vi "BMark_OpenWindow.vi"(6 "Graveyward Position Key":string="Eulogy.Graveyard.Position", 8 "Error In":errorcluster, 11 "Graveyard Window In":refnum<vi>) -> (0 "Error Out":errorcluster, 2 "Bounds":T1, 3 "Graveyward Window Out":refnum<vi>)   [LabVIEW 2018, in "Bookmark Manager.lvlib"]
uses:
  Bookmark Manager.lvlib
  <resource>/dialog/lvconfig.llb/LV Config Read String.vi
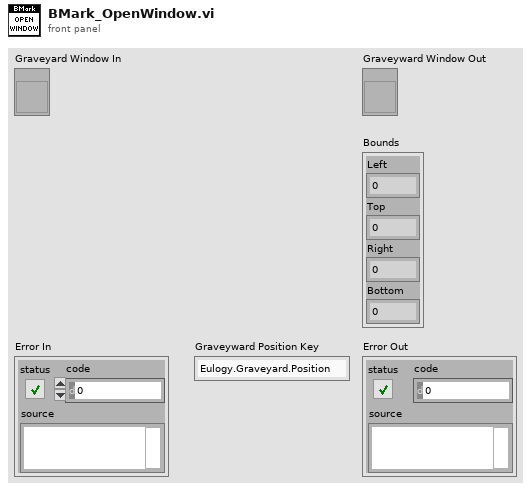
[diagram p1: front panel]
types:
  T1 = cluster{"Left":i16, "Top":i16, "Right":i16, "Bottom":i16}
  T2 = enum32{"Invalid", "Standard", "Closed", "Hidden", "Minimized", "Maximized"}
  T3 = typedef "LVAllMonitorsDisplayTypeDef.ctl" = cluster{"Bounds":cluster{"Left":i16, "Top":i16, "Right":i16, "Bottom":i16}, "Depth":i16}[]
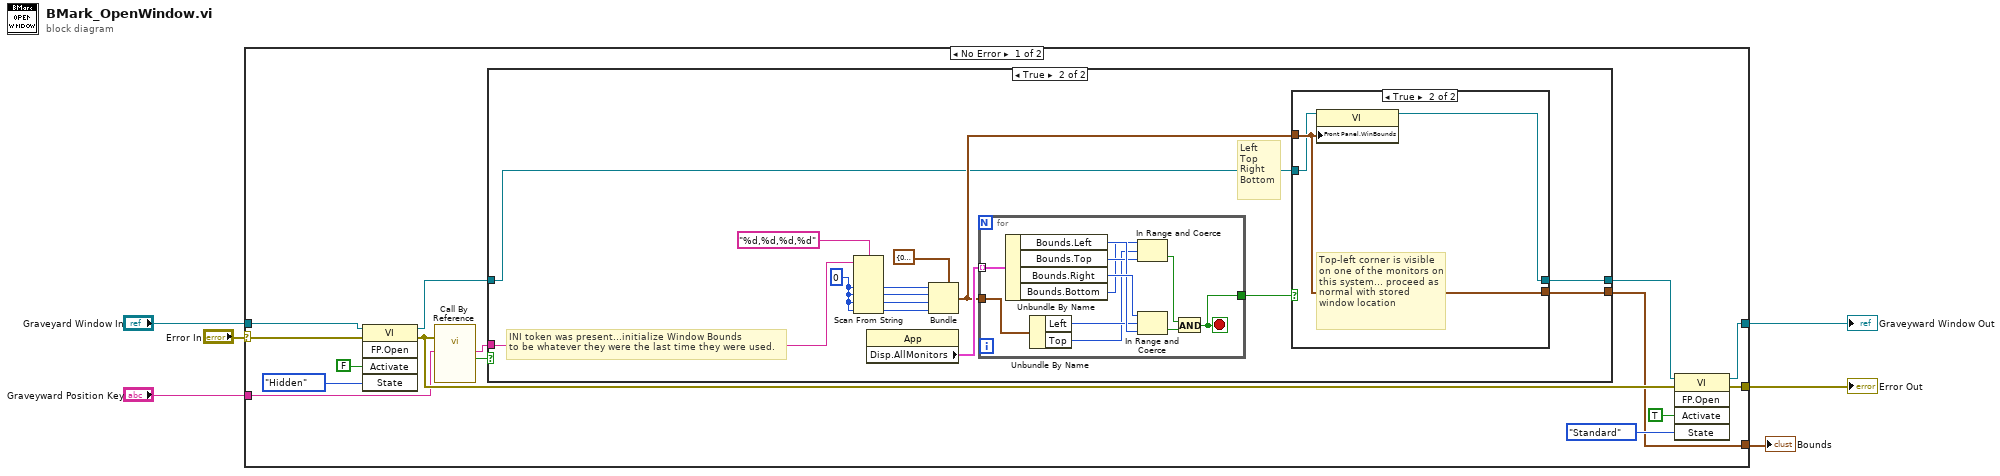
[diagram p0: block diagram]
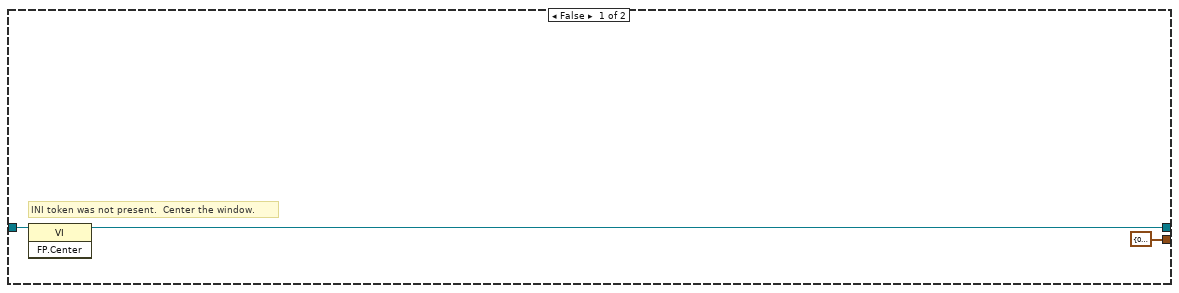
[diagram p2: hidden frame]
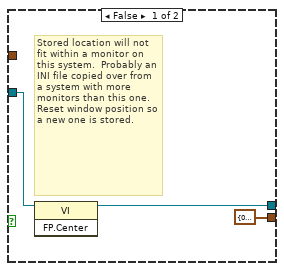
[diagram p3: hidden frame]
diagram:
  n1 = case shown="No Error" "Error In" {
    selector: "Error In" -> [w8 w57]
    tunnel: "Graveyard Window In" -> [w19 w56]
    tunnel: [w12 w56] -> w5
    tunnel: [w11 w57] -> w4
    tunnel: [w9 _] -> w3
    tunnel: "Graveyward Position Key" -> [w7 _]
    frame No Error {
      n2 = invoke class="VI" method="FP.Open"(reference=w19, error in=w8, "Activate"=FALSE ("Activate?"), "State"=T2."Hidden") -> (reference out=w14:refnum<vi>, error out=w10:errorcluster)  [unwired: 1 in, 3 out]
      n3 = call-by-ref "?"(error in=w10, "key"=w7) -> ("found?"=w15:bool, "value"=w16:string)  [unwired: 5 in, 3 out]
      n4 = case shown="True" w15 {
        tunnel: [T1 {"Left"=0, "Top"=0, "Right"=0, "Bottom"=0} ("Front Panel.PanelBounds") w27] -> w9
        tunnel: w16 -> [_ w38]
        tunnel: w14 -> [w23 w26]
        tunnel: [w22 w25] -> w13
        frame False {
          # "INI token was not present.  Center the window."
          n5 = invoke class="VI" method="FP.Center"(reference=w23) -> (reference out=w22:refnum<vi>)  [unwired: 2 in, 2 out]
        }
        frame True {
          w36 = i16 0 ("default value 1")
          # "Left\nTop\nRight\nBottom"
          # "INI token was present...initialize Window Bounds\nto be whatever they were the last time they were used."
          n6 = Scan From String(format string="%d,%d,%d,%d", input string=w38, default 1=w36, default 2=w36, default 3=w36, default 4=w36) -> (output 1=w35:i16, output 2=w34:i16, output 3=w33:i16, output 4=w32:i16)  [unwired: 2 in, 3 out]
          n7 = property class="App"() -> ("Disp.AllMonitors"=w30:T3)  [unwired: 2 in, 2 out]
          n8 = Bundle(cluster=T1 {"Left"=0, "Top"=0, "Right"=0, "Bottom"=0} ("Front Panel.PanelBounds"), "Left"=w35, "Top"=w34, "Right"=w33, "Bottom"=w32) -> (w29:T1)
          n9 = for {
            tunnel: w30 -> [w55] mode=indexing
            tunnel: w29 -> [w54]
            tunnel: [w45] -> w28
            stop <- w45 stop-if-true
            n10 = Unbundle By Name(w55) -> ("Bounds.Left"=w52:i16, "Bounds.Top"=w50:i16, "Bounds.Right"=w53:i16, "Bounds.Bottom"=w49:i16)
            n11 = Unbundle By Name(w54) -> ("Left"=w51:i16, "Top"=w48:i16)
            n12 = In Range and Coerce(upper limit=w49, x=w48, lower limit=w50) -> (In Range?=w47:bool)  [unwired: 1 out]
            n13 = In Range and Coerce(upper limit=w53, x=w51, lower limit=w52) -> (In Range?=w46:bool)  [unwired: 1 out]
            n14 = And(x=w47, y=w46) -> (x .and. y?=w45:bool)
          }
          n15 = case shown="True" w28 {
            tunnel: w29 -> [_ w44]
            tunnel: [T1 {"Left"=0, "Top"=0, "Right"=0, "Bottom"=0} ("Front Panel.PanelBounds") w44] -> w27
            tunnel: w26 -> [w40 w43]
            tunnel: [w39 w42] -> w25
            frame False {
              # "Stored location will not fit within a monitor on this system.  Probably an INI file copied over from a system with more monitors than this one.  Reset window position so a new one is stored."
              n16 = invoke class="VI" method="FP.Center"(reference=w40) -> (reference out=w39:refnum<vi>)  [unwired: 2 in, 2 out]
            }
            frame True {
              # "Top-left corner is visible on one of the monitors on this system... proceed as normal with stored window location"
              n17 = property class="VI"(reference=w43, "Front Panel.WinBounds"=w44) -> (reference out=w42:refnum<vi>)  [unwired: 1 in, 1 out]
            }
          }
        }
      }
      n18 = invoke class="VI" method="FP.Open"(reference=w13, error in=w10, "Activate"=TRUE ("Activate?"), "State"=T2."Standard") -> (reference out=w12:refnum<vi>, error out=w11:errorcluster)  [unwired: 1 in, 3 out]
    }
    frame Error {
    }
  }
  "Error Out" <- w4
  "Graveyward Window Out" <- w5
  "Bounds" <- w3
